vi "xianshi.vi"(0 "心率":u32) -> (1 "标题":string, 2 "心率转盘":dbl(knob) scale=0.0..150.0 scale format="%#_15g", 3 "心率":u32 caption="Numeric")   [LabVIEW 2016]
panel:
  # "心率测试"
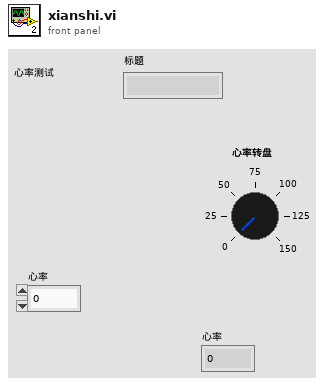
[diagram p1: front panel]
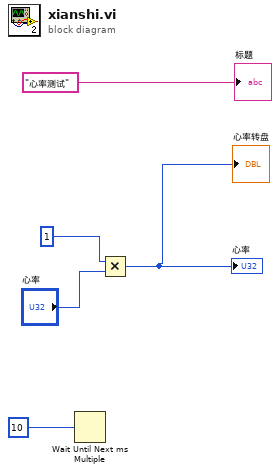
[diagram p0: block diagram]
diagram:
  n1 = Wait Until Next ms Multiple(millisecond multiple=10) -> ()  [unwired: 1 out]
  n2 = Multiply(x=1, y="心率") -> (x*y=→"心率转盘" →"心率":u32)
  "标题" <- "心率测试"
